vi "winch down_r2.vi"() -> ()   [LabVIEW 2015]
uses:
  <vilib>/myRIO/Instrument Drivers/Onboard IO/AI/typedefs/AI Reference.ctl
  <vilib>/myRIO/Common/Instrument Driver Framework/Utilities/typedefs/myRIO Generic Hardware Reference.ctl
  <vilib>/myRIO/Common/Instrument Driver Framework/Utilities/typedefs/Hardware Version Enum.ctl
  <vilib>/myRIO/Common/Instrument Driver Framework/Utilities/typedefs/myRIO v1.0 Reference.ctl
  <vilib>/myRIO/Common/Instrument Driver Framework/Utilities/typedefs/Generic FPGA Reference.ctl
  <vilib>/myRIO/Common/Instrument Driver Framework/myRIO v1.0/AI/typedefs/AI Channels List.ctl
  <vilib>/myRIO/Common/Instrument Driver Framework/myRIO v1.0/AI/typedefs/AI Channels Enum.ctl
  <vilib>/myRIO/Common/Instrument Driver Framework/Utilities/typedefs/Analog Scaling Constants List.ctl
  <vilib>/myRIO/Common/Instrument Driver Framework/Utilities/typedefs/Analog Scaling Constants.ctl
  <vilib>/userdefined/High Color/nirio_resource_hc.ctl
  <vilib>/myRIO/Instrument Drivers/Onboard IO/PWM/typedefs/PWM Reference.ctl
  <vilib>/myRIO/Common/Instrument Driver Framework/myRIO v1.0/PWM/typedefs/PWM Channels Enum.ctl
  <vilib>/myRIO/Instrument Drivers/Onboard IO/PWM/typedefs/PWM Configuration.ctl
  <vilib>/myRIO/Common/Instrument Driver Framework/Utilities/vis/Is FPGA Ref Available.vi
  <vilib>/myRIO/Common/Instrument Driver Framework/myRIO v1.0/AI/vis/myRIO v1.1 Open AI.vi
  <vilib>/myRIO/Instrument Drivers/Onboard IO/AI/vis/Read.vi
  <vilib>/myRIO/Common/Instrument Driver Framework/myRIO v1.0/PWM/vis/myRIO v1.1 Open PWM.vi
  <vilib>/myRIO/Instrument Drivers/Onboard IO/PWM/vis/Set Duty Cycle and Frequency.vi
  <vilib>/myRIO/Common/Instrument Driver Framework/Utilities/vis/Validate Channels.vi
  <vilib>/myRIO/Common/Instrument Driver Framework/myRIO v1.0/AI/vis/myRIO v1.0 Reserve AI.vi
  <vilib>/myRIO/Common/Instrument Driver Framework/myRIO v1.0/PWM/vis/myRIO v1.0 Reserve PWM.vi
  <vilib>/myRIO/Common/Instrument Driver Framework/myRIO v1.0/AI/vis/myRIO v1.0 Build MUX Configuration AI.vi
  <vilib>/myRIO/Common/Instrument Driver Framework/myRIO v1.0/Resource Manager/vis/myRIO v1.0 Reserve Channel List.vi
  <vilib>/myRIO/Common/Instrument Driver Framework/myRIO v1.0/PWM/vis/myRIO v1.0 Build MUX Configuration PWM.vi
  <vilib>/myRIO/Common/Instrument Driver Framework/myRIO v1.0/Resource Manager/vis/myRIO v1.0 Reserve Channel.vi
  <vilib>/myRIO/Common/Instrument Driver Framework/myRIO v1.0/Resource Manager/vis/myRIO v1.0 Unreserve Channel.vi
  <vilib>/myRIO/Common/Instrument Driver Framework/myRIO v1.0/Resource Manager/vis/myRIO v1.0 Create Configuration List.vi
  <vilib>/myRIO/Common/Instrument Driver Framework/myRIO v1.0/Resource Manager/vis/myRIO v1.0 Build Mutex Name.vi
  <vilib>/Utility/VariantDataType/GetNumericInfo.vi
  <vilib>/Utility/error.llb/Error Cluster From Error Code.vi
  <vilib>/myRIO/Common/Instrument Driver Framework/myRIO v1.0/myRIO v1.1 Open.vi
  <vilib>/myRIO/Common/Instrument Driver Framework/myRIO v1.0/AI/vis/myRIO v1.0 Get Scaling Constants AI.vi
  <vilib>/myRIO/Common/Instrument Driver Framework/Utilities/vis/IO Manager.vi
  <vilib>/myRIO/Common/Instrument Driver Framework/Utilities/vis/Configuration Manager.vi
  <vilib>/myRIO/Common/Instrument Driver Framework/myRIO v1.0/myRIO v1.0 Close.vi
  <vilib>/myRIO/Common/Instrument Driver Framework/myRIO v1.0/AI/vis/myRIO v1.0 Read AI.vi
  <vilib>/myRIO/Common/Instrument Driver Framework/myRIO v1.0/Resource Manager/vis/myRIO v1.0 Configure IO.vi
  <vilib>/myRIO/Common/Instrument Driver Framework/myRIO v1.0/PWM/vis/myRIO v1.0 Write PWM.vi
  <vilib>/myRIO/Express VI/Onboard IO/AI/AI Express VI.xnode
  <vilib>/myRIO/Instrument Drivers/Onboard IO/AI/vis/myRIO AI Open.xnode
  <vilib>/myRIO/Express VI/Onboard IO/PWM/PWM Express VI.xnode
  <vilib>/myRIO/Instrument Drivers/Onboard IO/PWM/vis/myRIO PWM Open.xnode
  <vilib>/myRIO/Instrument Drivers/Onboard IO/PWM/PWM.lvlib
  <vilib>/myRIO/Instrument Drivers/Onboard IO/AI/AI.lvlib
panel:
  out "rpm":dbl
  out "going up?":bool
  out "position 2":dbl
  out "position 1":dbl
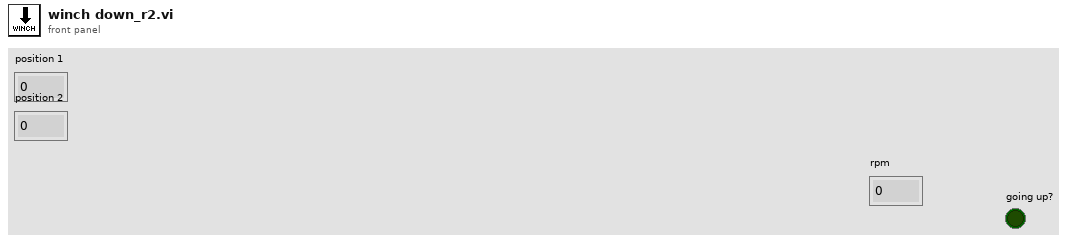
[diagram p1: front panel]
types:
  T1 = typedef "AI.lvlib/AI Reference.ctl" = cluster{"myRIO Reference":T2, "AI Channels List":T6, "AI Scaling Constants List":T8}
  T2 = typedef "myRIO Generic Hardware Reference.ctl" = cluster{"myRIO Model":T3, "myRIO Hardware Reference":T4}
  T3 = typedef "Hardware Version Enum.ctl" = enum16{"Unknown", "myRIO-1900", "myRIO-1950", "roboRIO"}
  T4 = typedef "myRIO v1.0 Reference.ctl" = cluster{"Generic FPGA Reference":T5, "Allow multiple opens":bool}
  T5 = typedef "Generic FPGA Reference.ctl" = refnum<k20>
  T6 = typedef "AI Channels List.ctl" = T7[]
  T7 = typedef "AI Channels Enum.ctl" = enum16{"Not Connected", "AudioIn/Left", "AudioIn/Right", "C/AI0", "C/AI1", "A/AI0", "A/AI1", "A/AI2", "A/AI3", "B/AI0", "B/AI1", "B/AI2", "B/AI3", "AI/AI0", "AI/AI1", "AI/AI2", "AI/AI3"}
  T8 = typedef "Analog Scaling Constants List.ctl" = T9[]
  T9 = typedef "Analog Scaling Constants.ctl" = cluster{"LSB Weight (Volts)":dbl, "Offset (Volts)":dbl, "Signed?":bool}
  T10 = typedef "nirio_resource_hc.ctl" = tag
  T11 = typedef "PWM.lvlib/PWM Reference.ctl" = cluster{"myRIO Reference":T2, "PWM Channels Enum":T12, "PWM Configuration":T13}
  T12 = typedef "PWM Channels Enum.ctl" = enum16{"Not Connected", "C/PWM0", "C/PWM1", "A/PWM0", "A/PWM1", "A/PWM2", "B/PWM0", "B/PWM1", "B/PWM2", "PWM/PWM0", "PWM/PWM1", "PWM/PWM2", "PWM/PWM3", "PWM/PWM4", "PWM/PWM5", "PWM/PWM6", "PWM/PWM7", "PWM/PWM8", "PWM/PWM9"}
  T13 = typedef "PWM.lvlib/PWM Configuration.ctl" = cluster{"Frequency":dbl, "Duty Cycle":dbl}
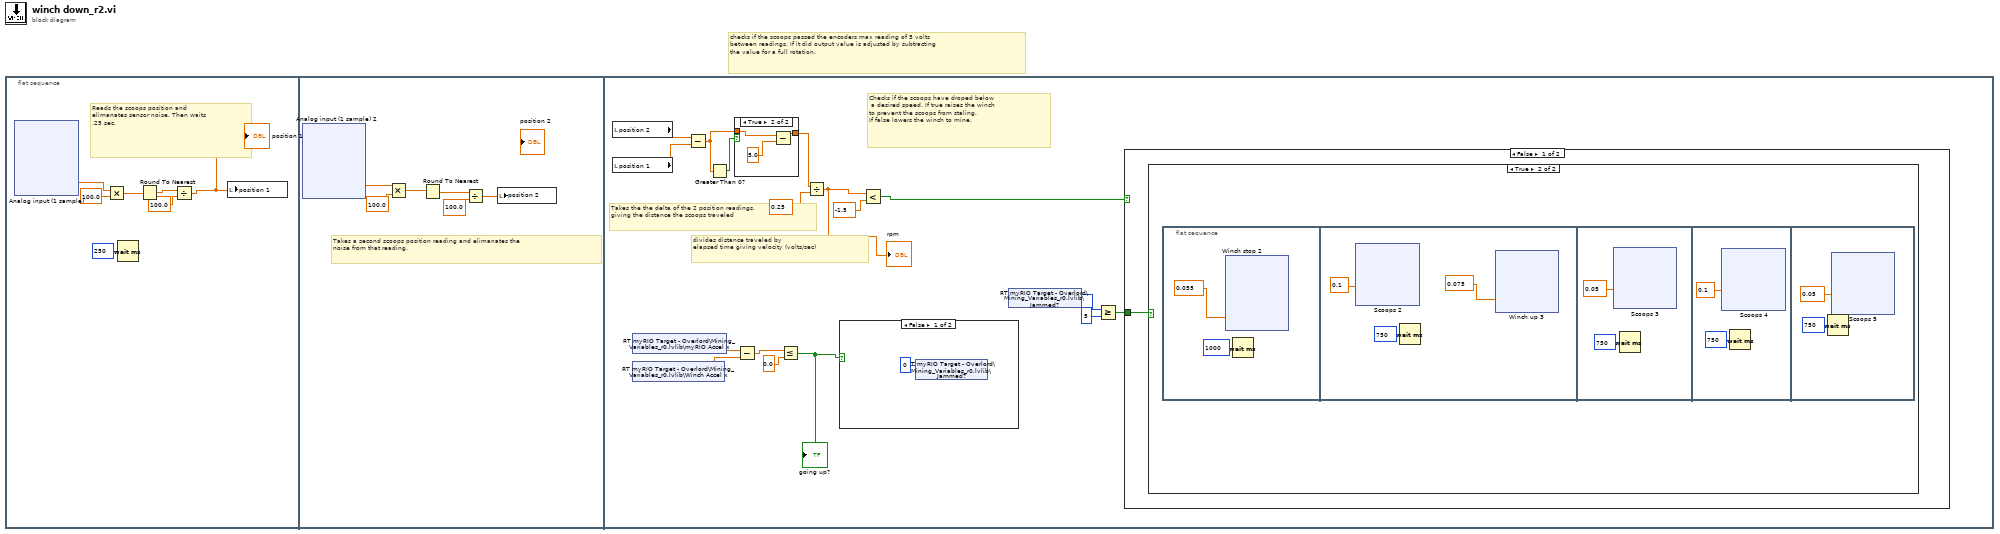
[diagram p0: block diagram]
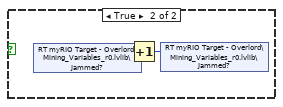
[diagram p2: hidden frame]
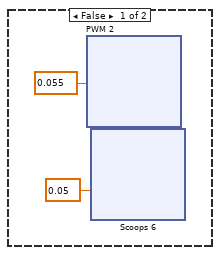
[diagram p3: hidden frame]
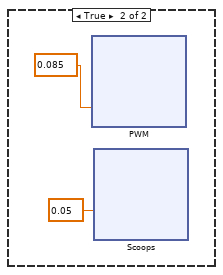
[diagram p4: hidden frame]
diagram:
  # "checks if the scoops passed the encoders max reading of 5 volts\nbetween readings. If it did output value is adjusted by subtracting \nthe value for a full rotation."
  n1 = flat-sequence {
    frame #0 {
      # "Reads the scoops position and \nelimanates sensor noise. Then waits\n.25 sec."
      n2 = xnode "Analog input (1 sample)"() -> ("A/AI1 (Pin 5)"=w5:dbl)  [unwired: 1 in, 1 out]
      n3 = Multiply(x=w5, y=100.0) -> (x*y=w4:dbl)
      n4 = Wait (ms)(milliseconds to wait=u32 250) -> ()  [unwired: 1 out]
      n5 = Round To Nearest(number=w4) -> (nearest integer value=w3:dbl)
      n6 = Divide(x=w3, y=100.0) -> (x/y=w1:dbl)
      "position 1" <- w1
      n7 = local write "position 1"(w1) -> ()
    }
    frame #1 {
      # "Takes a second scoops position reading and elimanates the \nnoise from that reading."
      n8 = xnode "Analog input (1 sample) 2"() -> ("A/AI1 (Pin 5)"=w47:dbl)  [unwired: 1 in, 1 out]
      n9 = Multiply(x=w47, y=100.0) -> (x*y=w48:dbl)
      n10 = Round To Nearest(number=w48) -> (nearest integer value=w49:dbl)
      n11 = Divide(x=w49, y=100.0) -> (x/y=w50:dbl)
      n12 = local write "position 2"(w50) -> ()
    }
    frame #2 {
      # "Checks if the scoops have droped below\n a desired speed. If true raises the winch \nto prevent the scoops from staling.\nIf false lowers the winch to mine."
      # "divides distance traveled by \nelapsed time giving velocity (volts/sec)"
      # "Takes the the delta of the 2 position readings.\ngiving the distance the scoops traveled"
      n13 = local read "position 2"() -> (w104:dbl)
      n14 = local read "position 1"() -> (w103:dbl)
      n15 = shared-variable "RT myRIO Target - Overlord\\Mining_Variables_r0.lvlib\\myRIO Accel x"() -> (w95:dbl)  [unwired: 1 in, 1 out]
      n16 = shared-variable "RT myRIO Target - Overlord\\Mining_Variables_r0.lvlib\\Winch Accel x"() -> (w94:dbl)  [unwired: 1 in, 1 out]
      n17 = Subtract(x=w104, y=w103) -> (x-y=w99:dbl)
      n18 = Greater Than 0?(x=w99) -> (x > 0?=w101:bool)
      n19 = case shown="True" w101 {
        tunnel: [w474 w477] -> w100
        tunnel: w99 -> [w474 w476]
        frame False {
        }
        frame True {
          n20 = Subtract(x=w476, y=5.0) -> (x-y=w477:dbl)
        }
      }
      n21 = Subtract(x=w95, y=w94) -> (x-y=w93:dbl)
      n22 = Less Or Equal?(x=w93, y=0.0) -> (x <= y?=w91:bool)
      "going up?" <- w91
      n23 = Divide(x=w100, y=0.25) -> (x/y=w96:dbl)
      "rpm" <- w96
      n24 = case shown="False" w91 {
        frame False {
          n25 = shared-variable "RT myRIO Target - Overlord\\Mining_Variables_r0.lvlib\\Jammed?"(u16 0 ("Jammed?")) -> ()  [unwired: 1 in, 1 out]
        }
        frame True {
          n26 = shared-variable "RT myRIO Target - Overlord\\Mining_Variables_r0.lvlib\\Jammed?"() -> (w107:u16)  [unwired: 1 in, 1 out]
          n27 = Increment(x=w107) -> (x+1=w106:u16)
          n28 = shared-variable "RT myRIO Target - Overlord\\Mining_Variables_r0.lvlib\\Jammed?"(w106) -> ()  [unwired: 1 in, 1 out]
        }
      }
      n29 = Less?(x=w96, y=-1.5) -> (x < y?=w97:bool)
      n30 = shared-variable "RT myRIO Target - Overlord\\Mining_Variables_r0.lvlib\\Jammed?"() -> (w90:u16)  [unwired: 1 in, 1 out]
      n31 = Greater Or Equal?(x=w90, y=u16 5) -> (x >= y?=w88:bool)
      n32 = case shown="False" w97 {
        tunnel: w88 -> [w108 _]
        frame False {
          n33 = case shown="True" w108 {
            frame False {
              n34 = xnode "PWM 2"("Duty Cycle"=0.055) -> ()  [unwired: 1 in, 1 out]
              n35 = xnode "Scoops 6"("Duty Cycle"=0.05) -> ()  [unwired: 1 in, 1 out]
            }
            frame True {
              n36 = flat-sequence {
                frame #0 {
                  n37 = xnode "Winch stop 2"("Duty Cycle"=0.055) -> ()  [unwired: 1 in, 1 out]
                  n38 = Wait (ms)(milliseconds to wait=u32 1000) -> ()  [unwired: 1 out]
                }
                frame #1 {
                  n39 = xnode "Scoops 2"("Duty Cycle"=0.1) -> ()  [unwired: 1 in, 1 out]
                  n40 = Wait (ms)(milliseconds to wait=u32 750) -> ()  [unwired: 1 out]
                  n41 = xnode "Winch up 3"("Duty Cycle"=0.075) -> ()  [unwired: 1 in, 1 out]
                }
                frame #2 {
                  n42 = xnode "Scoops 3"("Duty Cycle"=0.05) -> ()  [unwired: 1 in, 1 out]
                  n43 = Wait (ms)(milliseconds to wait=u32 750) -> ()  [unwired: 1 out]
                }
                frame #3 {
                  n44 = xnode "Scoops 4"("Duty Cycle"=0.1) -> ()  [unwired: 1 in, 1 out]
                  n45 = Wait (ms)(milliseconds to wait=u32 750) -> ()  [unwired: 1 out]
                }
                frame #4 {
                  n46 = Wait (ms)(milliseconds to wait=u32 750) -> ()  [unwired: 1 out]
                  n47 = xnode "Scoops 5"("Duty Cycle"=0.05) -> ()  [unwired: 1 in, 1 out]
                }
              }
            }
          }
        }
        frame True {
          n48 = xnode "PWM"("Duty Cycle"=0.085) -> ()  [unwired: 1 in, 1 out]
          n49 = xnode "Scoops"("Duty Cycle"=0.05) -> ()  [unwired: 1 in, 1 out]
        }
      }
    }
  }
